vi "Calculate Elo Ratings.vi"(11 "Names":T1[](array[typedef])) -> (0 "New Ratings":string[](array[string]), 1 "Names Out":string[](array[string]), 3 "Rating 2D Array":string[][](array[string]))   [LabVIEW 2014]
uses:
  User Score Update.ctl
  <vilib>/Utility/file.llb/Read From Spreadsheet File (string).vi
  <vilib>/Utility/file.llb/Write To Spreadsheet File (string).vi
panel:
  out "R Values":dbl[](array[numeric])
  out "Old":T1[](array[typedef])
  in  "Path":path=path "C:/Users/Justin/Desktop/LabVIEW-Rank/LabView Contests/Results/Elo_Ratings.csv"
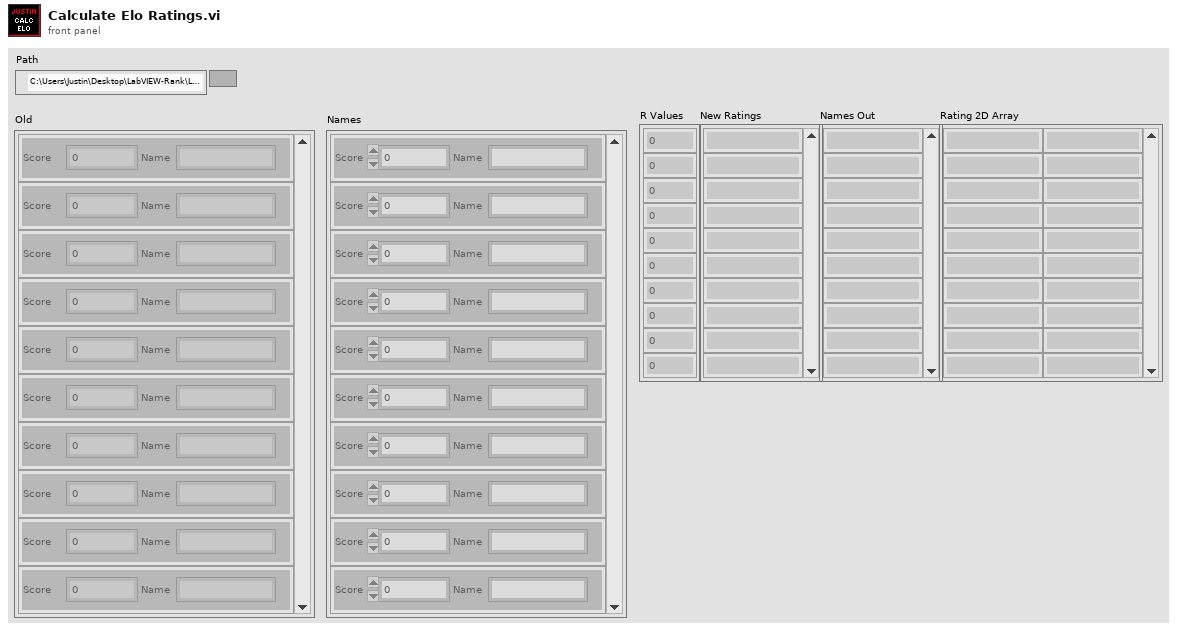
[diagram p1: front panel]
types:
  T1 = typedef "User Score Update.ctl" = cluster{"Score":dbl, "Name":string}
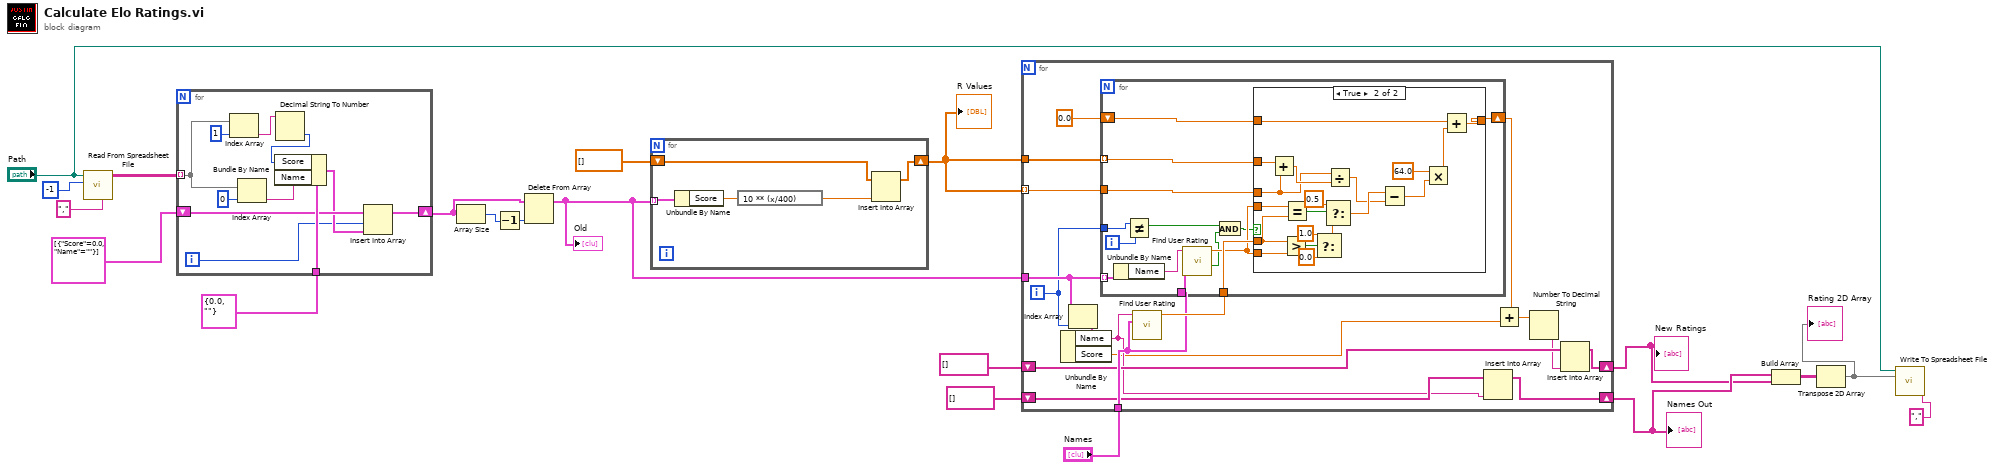
[diagram p0: block diagram]
diagram:
  n1 = call-poly <vilib>:"Read From Spreadsheet File.vi"("delimiter (\\t)"="," ("delimiter (\\t)"), "number of rows (all:-1)"=-1, "file path (dialog if empty)"="Path") -> ("all rows"=w18:string[][])  [unwired: 4 in, 4 out]
  n2 = for {
    tunnel: w18 -> [w28] mode=indexing
    shift-right: [w22] -> w13
    shift-left: T1[] [{"Score"=0.0, "Name"=""}] ("Score Ctl") -> [w24]
    tunnel: T1 {"Score"=0.0, "Name"=""} ("Score Update") -> [w25]
    i -> [w21]
    n3 = Index Array(array=w28, index=1) -> (element=w26:string)
    n4 = Index Array(array=w28, index=0) -> (element=w30:string)
    n5 = Decimal String To Number(string=w26) -> (number=w27:i32)  [unwired: 2 in, 1 out]
    n6 = Bundle By Name(cluster=w25, "Score"=w27, "Name"=w30) -> (w23:T1)
    n7 = Insert Into Array(array=w24, index=w21, new element=w23) -> (w22:T1[])
  }
  n8 = Array Size(array=w13) -> (size(s)=w14:i32)
  n9 = Decrement(x=w14) -> (x-1=w15:i32)
  n10 = Delete From Array(array=w13, index=w15) -> (array with subset deleted=w10:T1[])  [unwired: 1 in, 1 out]
  "Old" <- w10
  n11 = for {
    tunnel: w10 -> [w36] mode=indexing
    shift-right: [w32] -> w11
    shift-left: dbl[] [] -> [w33]
    n12 = Unbundle By Name(w36) -> ("Score"=w35:dbl)
    n13 = expression code="10 ** (x/400)"(w35) -> (w34:dbl)
    n14 = Insert Into Array(array=w33, new element=w34) -> (w32:dbl[])  [unwired: 1 in]
  }
  "R Values" <- w11
  n15 = for {
    tunnel: w11 -> [w53]
    tunnel: w11 -> [w43] mode=indexing
    tunnel: w10 -> [w51]
    tunnel: "Names" -> [w47]
    shift-right: [w45] -> w2
    shift-left: string[] [] -> [w46]
    shift-right: [w40] -> w3
    shift-left: string[] [] -> [w42]
    i -> [w50]
    n16 = Index Array(array=w51, index=w50) -> (element=w49:T1)
    n17 = Unbundle By Name(w49) -> ("Name"=w41:string, "Score"=w39:dbl)
    n18 = call "Find User Rating.vi"("Names"=w47, "String"=w41) -> ("Score"=w48:dbl)  [unwired: 8 in, 1 out]
    n19 = for {
      tunnel: w53 -> [w63] mode=indexing
      tunnel: w43 -> [w62]
      shift-right: [w65] -> w44
      shift-left: 0.0 -> [w64]
      tunnel: w50 -> [w66]
      tunnel: w51 -> [w60] mode=indexing
      tunnel: w48 -> [w61]
      tunnel: w47 -> [w58]
      i -> [w67]
      n20 = Unbundle By Name(w60) -> ("Name"=w59:string)
      n21 = Not Equal?(x=w66, y=w67) -> (x != y?=w56:bool)
      n22 = call "Find User Rating.vi"("Names"=w58, "String"=w59) -> ("Found?"=w54:bool, "Score"=w57:dbl)  [unwired: 8 in]
      n23 = And(x=w56, y=w54) -> (x .and. y?=w55:bool)
      n24 = case shown="True" w55 {
        tunnel: [w68 w71] -> w65
        tunnel: w64 -> [w68 w69]
        tunnel: w63 -> [_ w83]
        tunnel: w62 -> [_ w84]
        tunnel: w61 -> [_ w76]
        tunnel: w57 -> [_ w75]
        tunnel: w57 -> [_ w74]
        frame False {
        }
        frame True {
          n25 = Add(x=w83, y=w84) -> (x+y=w87:dbl)
          n26 = Greater?(x=w76, y=w75) -> (0:w82:bool)
          n27 = Equal?(x=w74, y=w76) -> (x = y?=w86:bool)
          n28 = Select(t=1.0, s=w82, f=0.0) -> (s? t:f=w81:dbl)
          n29 = Select(t=0.5, s=w86, f=w81) -> (s? t:f=w78:dbl)
          n30 = Divide(x=w84, y=w87) -> (x/y=w77:dbl)
          n31 = Subtract(x=w78, y=w77) -> (x-y=w73:dbl)
          n32 = Multiply(x=64.0, y=w73) -> (x*y=w70:dbl)
          n33 = Add(x=w69, y=w70) -> (x+y=w71:dbl)
        }
      }
    }
    n34 = Insert Into Array(array=w42, new element=w41) -> (w40:string[])  [unwired: 1 in]
    n35 = Add(x=w44, y=w39) -> (x+y=w38:dbl)
    n36 = Number To Decimal String(number=w38) -> (decimal integer string=w37:string)  [unwired: 1 in]
    n37 = Insert Into Array(array=w46, new element=w37) -> (w45:string[])  [unwired: 1 in]
  }
  "Names Out" <- w3
  "New Ratings" <- w2
  n38 = Build Array(w3, w2) -> (w4:string[][])
  n39 = Transpose 2D Array(2D array=w4) -> (transposed array=w1:string[][])
  "Rating 2D Array" <- w1
  n40 = call-poly <vilib>:"Write To Spreadsheet File.vi"("delimiter (\\t)"="," ("delimiter (\\t)"), "2D data"=w1, "file path (dialog if empty)"="Path") -> ()  [unwired: 5 in, 1 out]
